vi "getT.vi"(3 "error in (no error)":errorcluster, 5 "Sensor":i32) -> (0 "error out":errorcluster, 2 "Temperatur":dbl)   [LabVIEW 2009]
panel:
  # "GPIB 24"
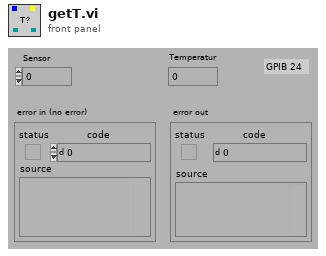
[diagram p1: front panel]
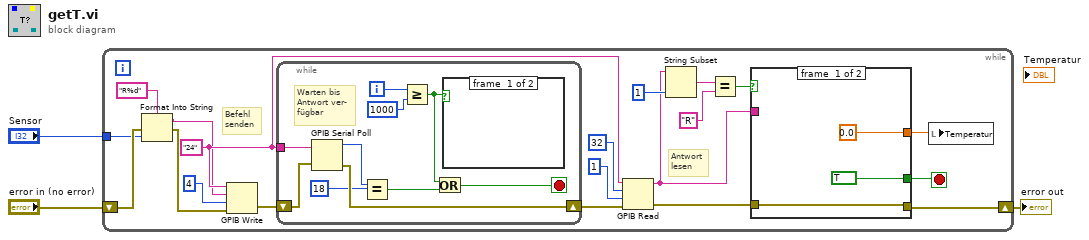
[diagram p0: block diagram]
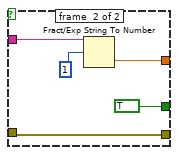
[diagram p2: hidden frame]
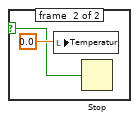
[diagram p3: hidden frame]
diagram:
  n1 = while {
    shift-right: [w10] -> w2
    shift-left: "error in (no error)" -> [w9]
    tunnel: "Sensor" -> [w8]
    stop <- w12 stop-if-true
    w18 = "24"
    # "Antwort\nlesen"
    # "Befehl\nsenden"
    n2 = Format Into String(format string="R%d", error in=w9, w8) -> (resulting string=w5:string, error out=w7:errorcluster)  [unwired: 1 in]
    n3 = GPIB Write(0:w18, 1:w5, 2:4, 3:w7) -> (6:w22:errorcluster)  [unwired: 1 in, 1 out]
    n4 = while {
      shift-right: [w40] -> w21
      shift-left: w22 -> [w41]
      tunnel: w18 -> [w39]
      i -> [w36]
      stop <- w34 stop-if-true
      # "Warten bis\nAntwort ver-\nfügbar"
      n5 = GPIB Serial Poll(0:w39, 1:w41) -> (2:w37:i16, 4:w40:errorcluster)  [unwired: 1 out]
      n6 = Equal?(x=w37, y=18) -> (x = y?=w33:bool)
      n7 = Greater Or Equal?(x=w36, y=1000) -> (x >= y?=w32:bool)
      n8 = Or(x=w32, y=w33) -> (x .or. y?=w34:bool)
      n9 = case shown="True" w32 {
        selector: w32 -> [_ w42]
        frame #0 {
        }
        frame #1 {
          n10 = local write "Temperatur"(0.0) -> ()
          n11 = Stop(stop? (T)=w42) -> ()
        }
      }
    }
    n12 = GPIB Read(0:w18, 1:32, 2:1, 3:w21) -> (5:w13:string, 7:w11:errorcluster)  [unwired: 1 in, 1 out]
    n13 = String Subset(string=w13, length (rest)=1) -> (substring=w16:string)  [unwired: 1 in]
    n14 = Equal?(x=w16, y="R") -> (x = y?=w14:bool)
    n15 = case shown="True" w14 {
      tunnel: w13 -> [_ w30]
      tunnel: [TRUE TRUE] -> w12
      tunnel: [w24 w28] -> w10
      tunnel: w11 -> [w24 w28]
      tunnel: [0.0 w27] -> w4
      frame #0 {
      }
      frame #1 {
        n16 = Fract/Exp String To Number(string=w30, offset=1) -> (number=w27:dbl)  [unwired: 2 in, 1 out]
      }
    }
    n17 = local write "Temperatur"(w4) -> ()
  }
  "error out" <- w2
